vi "sensor list.vi"() -> ()   [LabVIEW 2019]
uses:
  Main.lvclass
  Common/DataTypes/Sensor ranges--cluster.ctl
  Common/DataTypes/Sensor database record--cluster.ctl
  Common/DataTypes/Sensor LUT--cluster.ctl
panel:
  out "CurrSensor*":T1 {"last updated" format="%<%H:%M\n%d/%m/%Y>T"}
  in  "Main.lvclass":refnum<class "Main.lvclass">
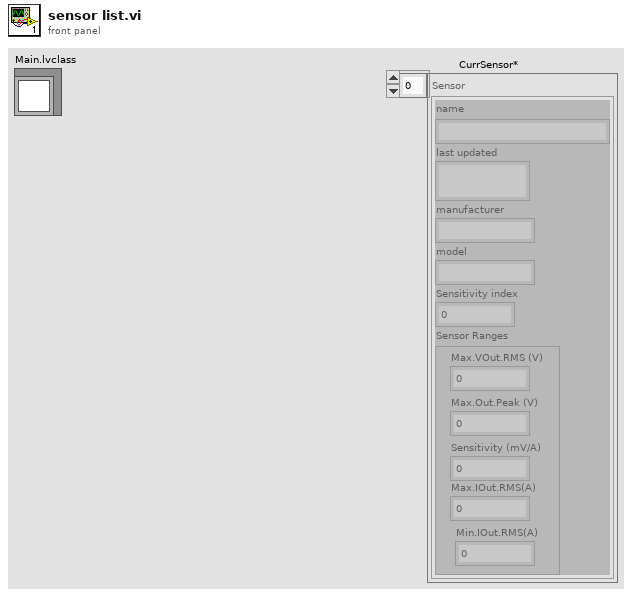
[diagram p1: front panel]
types:
  T1 = typedef "Sensor LUT--cluster.ctl" = T2[]
  T2 = typedef "Sensor database record--cluster.ctl" = cluster{"name":string, "last updated":timestamp, "manufacturer":string, "model":string, "Sensitivity index":dbl, "Sensor Ranges":T3}
  T3 = typedef "Sensor ranges--cluster.ctl" = cluster{"Max.VOut.RMS (V)":dbl, "Max.Out.Peak (V)":dbl, "Sensitivity (mV/A)":dbl, "Max.IOut.RMS(A)":dbl, "Min.IOut.RMS(A)":dbl}
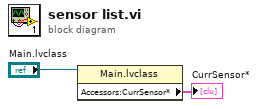
[diagram p0: block diagram]
diagram:
  n1 = property class="Main.lvclass"(reference="Main.lvclass") -> ("Accessors:CurrSensor*"=→"CurrSensor*":T1)  [unwired: 1 in, 2 out]
